vi "Test MFC Purge.vi"() -> ()   [LabVIEW 2013]
uses:
  Devices/Alicat/Session Based/Alicat Device.lvclass
  Reusable/Session APIs/File Access/Config Data/Config Session.ctl
  Reusable/Session APIs/File Access/Config Data/Config Data.lvclass
  Devices/Configurable Device/Configurable Device.lvclass/Configurable Device.ctl
  Devices/Alicat/Session Based/Alicat Device.lvclass/Alicat Device.ctl
  Devices/Alicat/Session Based/Data/MC/MC Data.lvclass
  Devices/Alicat/Session Based/Data/M/M data.lvclass
  Devices/Alicat/Session Based/Data/MC/MC Data.lvclass/MC Data.ctl
  Devices/Alicat/Session Based/Data/M/M data.lvclass/M data.ctl
  Devices/Alicat/Session Based/Data/MC/Accessors/Read P.vi
  Devices/Alicat/Session Based/Data/MC/Accessors/Read T.vi
  Devices/Alicat/Session Based/Data/M/Accessors/Read P.vi
  Devices/Alicat/Session Based/Data/M/Accessors/Read T.vi
  Devices/Configurable Device/Write Handle.vi
  Devices/Alicat/Session Based/Accessors/Write ID.vi
  Reusable/Data/Read measTime.vi
  Reusable/Session APIs/Serial/Serial Session.lvclass
  <userlib>/_Session Fwk/Session - Root.lvclass
panel:
  in  "Q0":dbl
  in  "stop":bool
  out "Acquisition Time":timestamp format="%<%H:%M:%S%2u>T"
  out "dataOut":cluster{"Accessors:P":sgl, "Accessors:T":sgl}(graph) caption="Alicat Data"
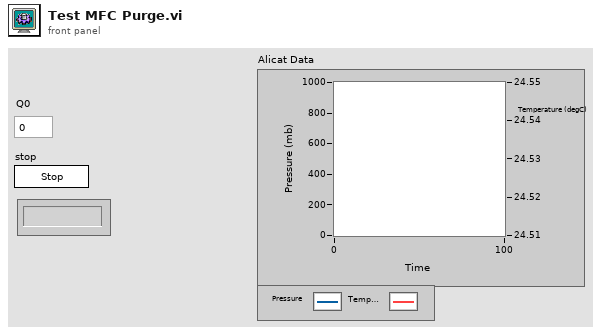
[diagram p1: front panel]
types:
  T1 = typedef "Config Data.lvclass/Config Session.ctl" = refnum<data-value>
  T2 = typedef "Session - Root.lvclass/Session Handle.ctl" = refnum<data-value>
  T3 = typedef "Serial Session.lvclass/Session Handle.ctl" = refnum<data-value>
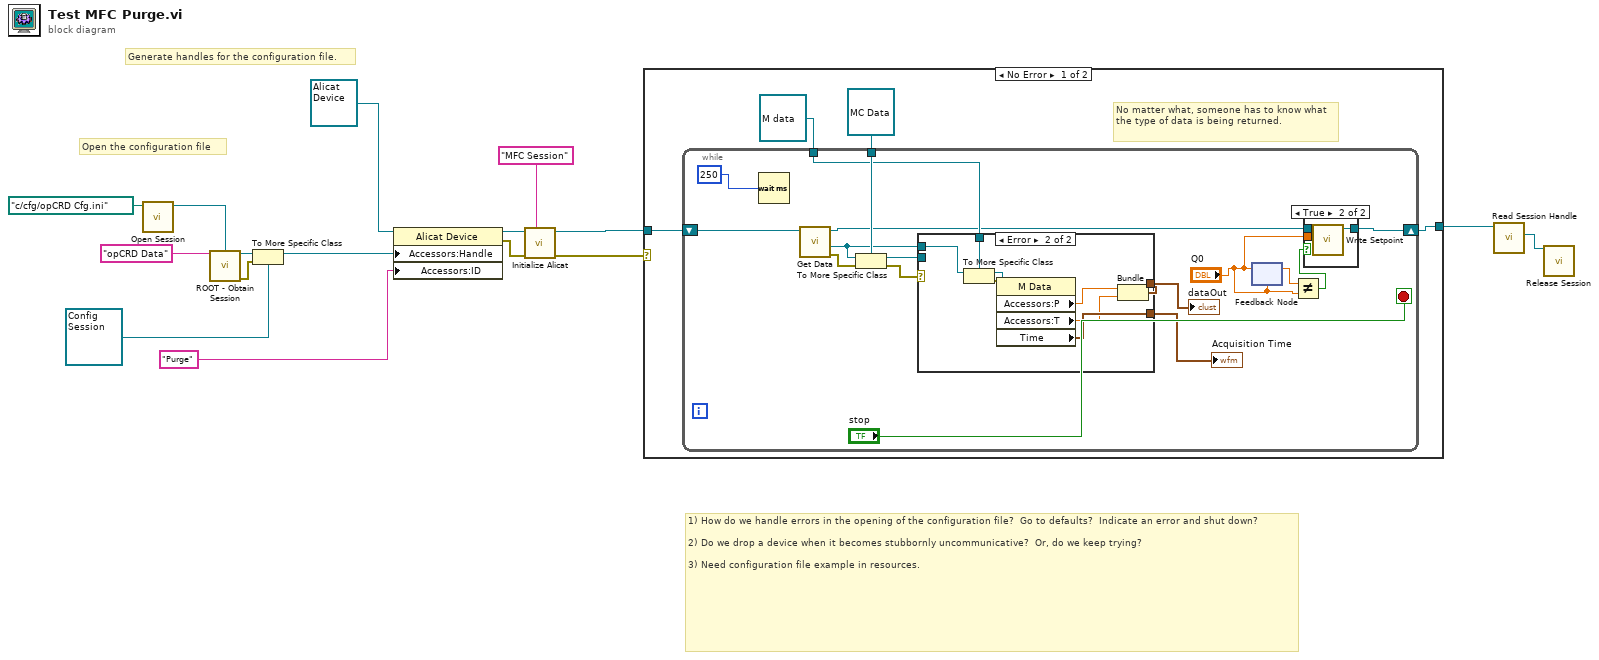
[diagram p0: block diagram]
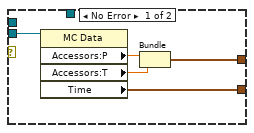
[diagram p3: hidden frame]
diagram:
  # "1) How do we handle errors in the opening of the configuration file?  Go to defaults?  Indicate an error and shut down?\n\n2) Do we drop a device when it becomes stubbornly uncommunicative?  Or, do we keep trying?\n\n3) Need configuration file example in resources."
  # "Open the configuration file"
  # "Generate handles for the configuration file."
  n1 = call "Open Session.vi"("Path"=path "c:/cfg/opCRD Cfg.ini") -> ("Config Data"=w11:refnum<class "Config Data.lvclass">)  [unwired: 9 in, 1 out]
  n2 = call <userlib>:"ROOT - Obtain Session.vi"("Session Name ()"="opCRD Data", "OBJ - Session"=w11) -> ("Session Handle"=w7:T2, "error out"=w6:errorcluster)  [unwired: 11 in, 1 out]
  n3 = To More Specific Class(target class=T1 refnum ("Session Handle"), reference=w7, error in=w6) -> (specific class reference=w9:T1)  [unwired: 1 out]
  n4 = property class="Alicat Device"(reference=refnum<class "Alicat Device.lvclass"> refnum ("Alicat Device in"), "Accessors:Handle"=w9, "Accessors:ID"="Purge") -> (reference out=w5:refnum<class "Alicat Device.lvclass">, error out=w4:errorcluster)  [unwired: 1 in]
  n5 = call "Initialize Alicat.vi"("Session Name ()"="MFC Session", "error in"=w4, "Alicat Device In"=w5) -> ("error out"=w15:errorcluster, "Alicat Device Out"=w14:refnum<class "Alicat Device.lvclass">)  [unwired: 7 in]
  n6 = case shown="No Error" w15 {
    tunnel: w14 -> [w19 w54]
    tunnel: [w17 w54] -> w1
    frame No Error {
      # "No matter what, someone has to know what the type of data is being returned."
      n7 = while {
        shift-right: [w24] -> w17
        shift-left: w19 -> [w36]
        tunnel: refnum<class "MC Data.lvclass"> refnum ("MC Data") -> [w35]
        tunnel: refnum<class "M data.lvclass"> refnum ("M Data") -> [w34]
        stop <- "stop" stop-if-true
        n8 = Wait (ms)(milliseconds to wait=250) -> ()  [unwired: 1 out]
        n9 = call "Get Data.vi"("Alicat Device in"=w36) -> ("error out"=w31:errorcluster, "Alicat Data out"=w28:refnum<class "Alicat Data.lvclass">, "Alicat Device out"=w25:refnum<class "Alicat Device.lvclass">)  [unwired: 7 in, 1 out]
        n10 = To More Specific Class(target class=w35, reference=w28, error in=w31) -> (specific class reference=w30:refnum<class "MC Data.lvclass">, error out=w29:errorcluster)
        n11 = case shown="Error" w29 {
          tunnel: w30 -> [w45 _]
          tunnel: [w42 w46] -> w32
          tunnel: [w41 w49] -> w27
          tunnel: w28 -> [_ w53]
          tunnel: w34 -> [_ w52]
          frame No Error {
            n12 = property class="MC Data"(reference=w45) -> ("Accessors:P"=w44:sgl, "Accessors:T"=w43:sgl, "Time"=w41:timestamp)  [unwired: 1 in, 2 out]
            n13 = Bundle("Accessors:P"=w44, "Accessors:T"=w43) -> (w42:cluster{"Accessors:P":sgl, "Accessors:T":sgl})  [unwired: 1 in]
          }
          frame Error {
            n14 = To More Specific Class(target class=w52, reference=w53) -> (specific class reference=w50:refnum<class "M data.lvclass">, error out=w51:errorcluster)  [unwired: 1 in]
            n15 = property class="M Data"(reference=w50, error in=w51) -> ("Accessors:P"=w48:sgl, "Accessors:T"=w47:sgl, "Time"=w49:timestamp)  [unwired: 2 out]
            n16 = Bundle("Accessors:P"=w48, "Accessors:T"=w47) -> (w46:cluster{"Accessors:P":sgl, "Accessors:T":sgl})  [unwired: 1 in]
          }
        }
        "dataOut" <- w32
        "Acquisition Time" <- w27
        n17 = feedback-in #1("Q0") -> ()
        n18 = feedback #1("Q0") -> (w23:dbl)
        n19 = Not Equal?(x=w23, y="Q0") -> (x != y?=w22:bool)
        n20 = case shown="True" w22 {
          tunnel: w25 -> [w37 w40]
          tunnel: [w37 w39] -> w24
          tunnel: "Q0" -> [_ w38]
          frame False {
          }
          frame True {
            n21 = call "Write Setpoint.vi"("Setpoint"=w38, "Alicat Device in"=w40) -> ("Alicat Device out"=w39:refnum<class "Alicat Device.lvclass">)  [unwired: 7 in, 2 out]
          }
        }
      }
    }
    frame Error {
    }
  }
  n22 = call "Read Session Handle.vi"("Alicat Device in"=w1) -> ("Session Handle"=w2:T3)  [unwired: 8 in, 2 out]
  n23 = call "Release Session.vi"("Session Handle"=w2) -> ()  [unwired: 14 in, 1 out]
